vi "H5Lget_val_by_idx (Soft).vi"(5 "Order":T2 items=["H5_ITER_UNKNOWN"=-1, "H5_ITER_INC"=0, "H5_ITER_DEC"=1], 6 "lapl_id":T4, 7 "Index Field":T1 items=["H5_INDEX_UNKNOWN"=-1, "H5_INDEX_NAME"=0, "H5_INDEX_CRT_ORDER"=1], 8 "error in (no error)":errorcluster, 9 "Index":u64, 10 "Name":string=".", 11 "Location Ref":T4) -> (0 "error out":errorcluster, 1 "Object Path":string, 3 "Location Ref out":T4, 4 "type":T3 items=["H5L_TYPE_ERROR"=-1, "H5L_TYPE_HARD"=0, "H5L_TYPE_SOFT"=1, "H5L_TYPE_EXTERNAL"=64, "H5L_TYPE_MAX"=255])   [LabVIEW 2017]
doc: "Retrieves value of the nth link in a group, according to the order within an index."
uses:
  <vilib>/UPVI/lvhdf5/library.llb/HDF5 Ref.ctl
  <vilib>/UPVI/lvhdf5/link.llb/H5L_type_t.ctl
  <vilib>/UPVI/lvhdf5/library.llb/H5_iter_order_t.ctl
  <vilib>/UPVI/lvhdf5/library.llb/H5_index_t.ctl
  <vilib>/UPVI/lvhdf5/error.llb/LVH5EMajorID.ctl
  <vilib>/UPVI/lvhdf5/error.llb/LVH5EMinorID.ctl
  <vilib>/UPVI/lvhdf5/error.llb/H5Epush_enum_enum.vi
panel:
  # "LVHDF5 Toolkit\nCopyright (c) 2005-2013 by Jason D. Sommerville\nCopyright (c) 2014-2015 by UPVI, LLC.\n\nThis use and distribution of this file is governed by the terms found in \nLICENSE.txt distributed with this toolkit and installed at\n <user.lib>\\_lvhdf5\\LICENSE.txt"
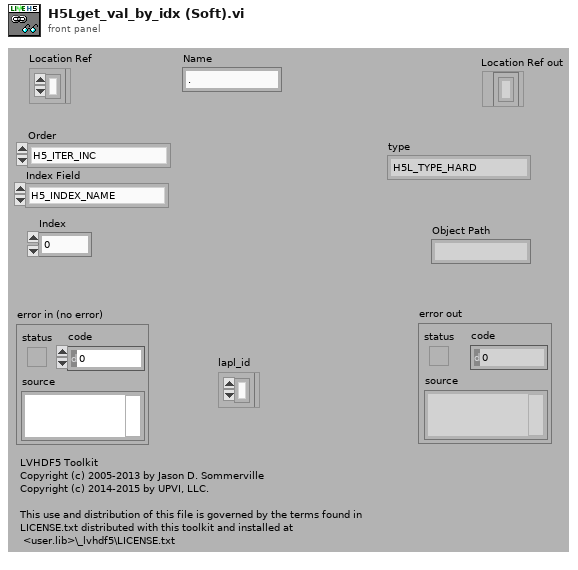
[diagram p1: front panel]
types:
  T1 = typedef "H5_index_t.ctl" = i32
  T2 = typedef "H5_iter_order_t.ctl" = i32
  T3 = typedef "H5L_type_t.ctl" = i32
  T4 = typedef "HDF5 Ref.ctl" = refnum<k1>
  T5 = typedef "LVH5EMinorID.ctl" = string
  T6 = typedef "LVH5EMajorID.ctl" = string
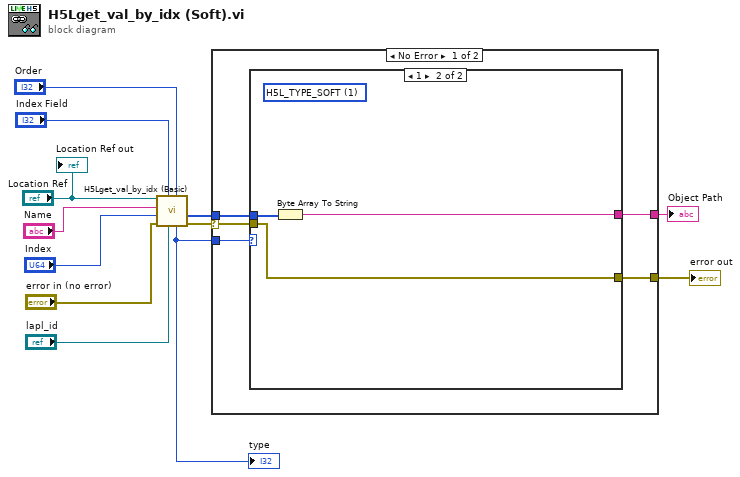
[diagram p0: block diagram]
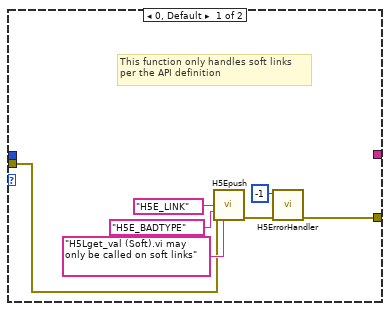
[diagram p2: hidden frame]
diagram:
  n1 = call <vilib>:"H5Lget_val_by_idx (Basic).vi"("Order"="Order", "lapl_id"="lapl_id", "Index Field"="Index Field", "error in (no error)"="error in (no error)", "Index"="Index", "Name"="Name", "Location Ref"="Location Ref") -> ("error out"=w8:errorcluster, "buffer"=w7:u8[], "type"=w6:T3)  [unwired: 1 in, 1 out]
  "type" <- w6
  n2 = case shown="No Error" w8 {
    selector: w8 -> [w14 w28]
    tunnel: w7 -> [w16 _]
    tunnel: w6 -> [w17 _]
    tunnel: [w15 _] -> w4
    tunnel: [w13 w28] -> w5
    frame No Error {
      n3 = case shown="1" w17 {
        tunnel: w16 -> [_ w27]
        tunnel: [_ w26] -> w15
        tunnel: w14 -> [w19 w25]
        tunnel: [w18 w25] -> w13
        frame 0, Default {
          # "This function only handles soft links\nper the API definition"
          n4 = call-poly <vilib>:"H5Epush.vi"("major_id"=T6 "H5E_LINK", "minor_id"=T5 "H5E_BADTYPE", "error in (no error)"=w19, "msg"="H5Lget_val (Soft).vi may only be called on soft links") -> ("error out"=w21:errorcluster)  [unwired: 10 in, 1 out]
          n5 = call <vilib>:"H5ErrorHandler.vi"("error in (no error)"=w21, "herr_t"=-1) -> ("error out"=w18:errorcluster)  [unwired: 3 in, 4 out]
        }
        frame 1 {
          (unwired) T3 1 items=["H5L_TYPE_ERROR"=-1, "H5L_TYPE_HARD"=0, "H5L_TYPE_SOFT"=1, "H5L_TYPE_EXTERNAL"=64, "H5L_TYPE_MAX"=255] ("type")
          n6 = Byte Array To String(unsigned byte array=w27) -> (string=w26:string)
        }
      }
    }
    frame Error {
    }
  }
  "error out" <- w5
  "Object Path" <- w4
  "Location Ref out" <- "Location Ref"
